vi "Select unique devices from File.vi"(11 "MaskFile":path=path "C:/Users/Flash/Desktop/Mask Files/SL066 Detector/SL066_mask_map_file_V3_align on D3000.csv") -> (3 "Device Array":string[](array[string]))   [LabVIEW 2012]
uses:
  <vilib>/Utility/file.llb/Read From Spreadsheet File (string).vi
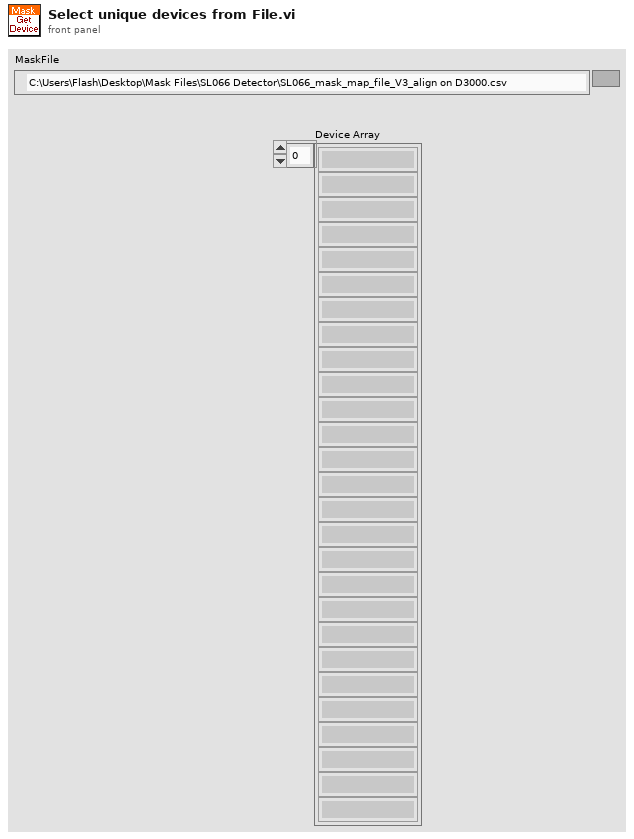
[diagram p1: front panel]
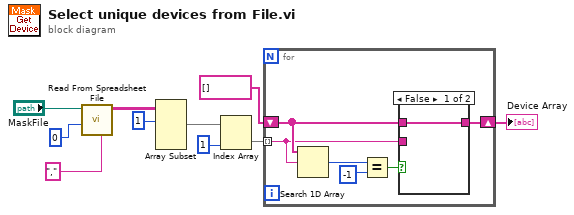
[diagram p0: block diagram]
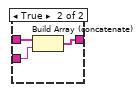
[diagram p2: hidden frame]
diagram:
  n1 = call-poly <vilib>:"Read From Spreadsheet File.vi"("delimiter (\\t)"="," ("delimiter (\\t)"), "start of read offset (chars.:0)"=0, "file path (dialog if empty)"="MaskFile") -> ("all rows"=w8:string[][])  [unwired: 4 in, 4 out]
  n2 = Array Subset(array=w8, index (row)=1 ("index")) -> (w6:string[][])  [unwired: 3 in]
  n3 = Index Array(array=w6, index (col)=1 ("disabled index (col)")) -> (element=w3:string[])  [unwired: 1 in]
  n4 = for {
    tunnel: w3 -> [w12] mode=indexing
    shift-right: [w16] -> w1
    shift-left: string[] [] ("subarray") -> [w15]
    n5 = Search 1D Array(1D array=w15, element=w12) -> (index of element=w14:i32)  [unwired: 1 in]
    n6 = Equal?(x=w14, y=-1) -> (x = y?=w11:bool)
    n7 = case shown="False" w11 {
      tunnel: [w17 w20] -> w16
      tunnel: w15 -> [w17 w19]
      tunnel: w12 -> [_ w18]
      frame False {
      }
      frame True {
        n8 = Build Array (concatenate)(w19, w18) -> (w20:string[])
      }
    }
  }
  "Device Array" <- w1
